vi "ALTS-2015 OPC Write Engine.vi"(8 "error in (no error)":errorcluster, 11 "Delay (ms)":u32=100) -> (0 "error out":errorcluster)   [LabVIEW 2013]
doc: "Copyright © 2005, Soliton Technologies.\nAll rights reserved."
uses:
  Controls/ALTS-2015 OPC Engine Main Options.ctl
  Controls/ALTS-2015 OPC Write Registers.ctl
  Controls/ALTS-2015 OPC Write Global Options.ctl
  Controls/ALTS-2015 OPC Global Options.ctl
  Controls/ALTS-2015 OPC Global Elements.ctl
  Globals/ALTS-2015 OPC Engine Globals.vi
  Controls/ALTS-2015 Safety Logic Cases.ctl
  SLL DAQ Engine/Software/Source Code/Controls/SLL DI Global Options.ctl
  SLL DAQ Engine/Software/Source Code/Controls/SLL List of Digital Inputs.ctl
panel:
  in  "OPC Write Registers":T1=enum."Serial_Flange_Size"
  out "Running Case":T2
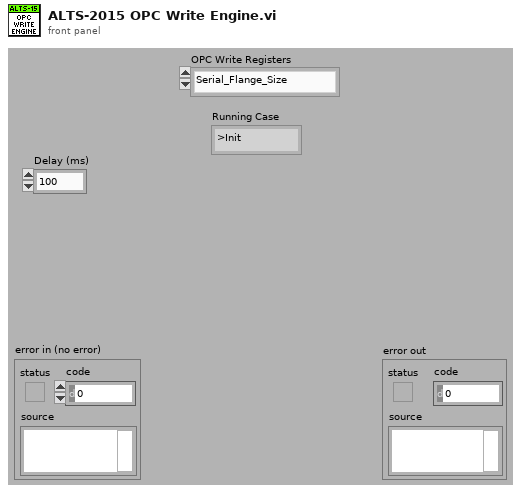
[diagram p1: front panel]
types:
  T1 = typedef "ALTS-2015 OPC Write Registers.ctl" = enum16{"Task_Available_for_Robot", "New_Serial", "Serial_Adapter_Size", "Serial_Displacement_Size", "Serial_Flange_Size", "Serial_Height", "Serial_LoadDecision", "Serial_CartInsert", "Test_Result", "Station_Number", "Rerun", "Invalid_SNo", "PC_ACK_Read_Tags", "No_Test"}
  T2 = typedef "ALTS-2015 OPC Engine Main Options.ctl" = enum16{">Init", ">Safe Mode", ">Poll", ">Error", ">Exit", ">Write", ">Read", ">Restart"}
  T3 = typedef "ALTS-2015 OPC Global Options.ctl" = enum16{"Init", "Write 1", "Read 1", "Write Array", "Read Array", "Clear"}
  T4 = typedef "ALTS-2015 OPC Write Global Options.ctl" = enum16{"Init", "Write Value", "Write Array", "Read Value", "Read Array", "Read All"}
  T5 = cluster{"Channel Order":i32[], "Connection ids":refnum<k13>[], "OPC Write Register Old Value":variant[]}
  T6 = enum16{"Read", "Write", "ReadWrite", "BufferedRead", "BufferedReadWrite"}
  T7 = typedef "ALTS-2015 OPC Global Elements.ctl" = enum16{"OPC - R Error", "OPC - W Error", "OPC - R Restart", "OPC - W Restart", "OPC - R Running", "OPC - W Running"}
  T8 = typedef "SLL List of Digital Inputs.ctl" = enum16{"MSSF", "MSSHC", "MSSMF", "MSSPRM", "MSSR", "PS01TS", "PX03TS", "PX04TS", "PX05TS", "PX06TS", "PX18TS", "READYTS"}
  T9 = typedef "SLL DI Global Options.ctl" = enum16{"Init", "Write Line", "Write Array", "Read Line", "Read Array", "Read Full Status", "Write Full Status"}
  T10 = typedef "ALTS-2015 Safety Logic Cases.ctl" = enum16{"Read S/W EStop", "Read H/W EStop", "Write S/W EStop", "Write H/W EStop", "Read S/W & H/W EStop"}
  T11 = typedef "ALTS-2015 INI Configuration Cluster.ctl" = cluster{"Application":cluster{"Rerun Count":i32, "Workorder No":string, "PLC Scanner":bool}, "Station Details":cluster{"Sensor Name 1":string, "Sensor Name 2":string, "Sensor Name 3":string, "Sensor Name 4":string, "Station1 Enable":bool, "Station2 Enable":bool, "Station3 Enable":bool, "Station4 Enable":bool}, "Database":cluster{"Database Connection Link":path, "Result Procedure":string, "User":string, "Password":string, "Prompt":bool, "Station 1 LT Result DB DSN Path":path, "Station 2 LT Result DB DSN Path":path, "Station 3 LT Result DB DSN Path":path, "Station 4 LT Result DB DSN Path":path, "AirLeakTestResult Procedure":string, "Serial Details Procedure":string}, "Simulation":cluster{"Simulate DAQ Hardware":bool, "Simulate Result DB Write":bool, "Simulate Scanner":bool, "Simulate OPC":bool, "Simulate Serial Details DB":bool, "Simulate Result DB":bool, "Simulate Scanner DB Path":path, "Simulate Serial Details DB Path":path, "Simulate Result DB Path":path}, "Barcode Scanner1":cluster{"Scanner IP":string, "Scanner Port":u16, "#Bytes to Read":i32, "Timeout_ms":i32}, "Barcode Scanner2":cluster{"Enabled?":bool, "Scanner IP":string, "Scanner Port":u16, "#Bytes to Read":i32}}
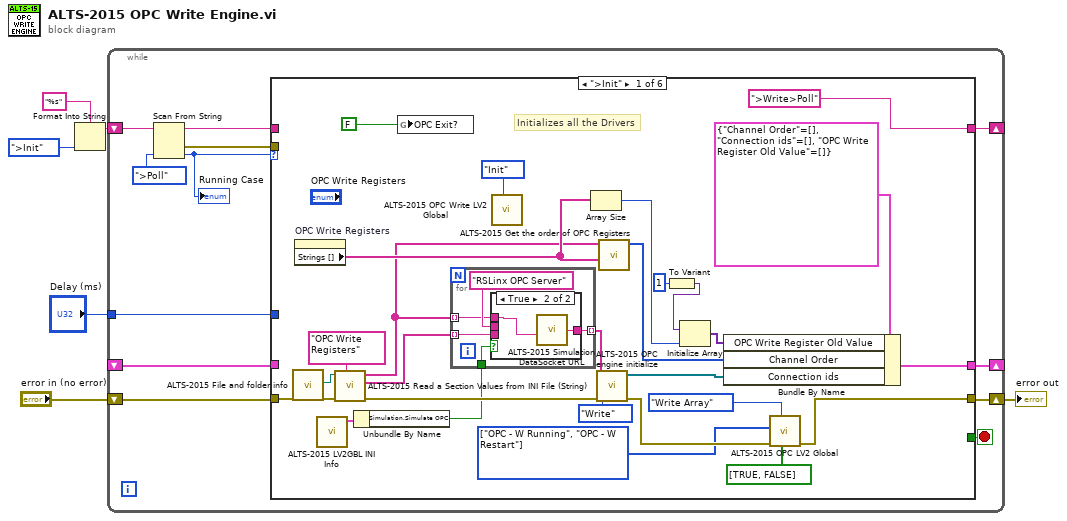
[diagram p0: block diagram]
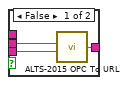
[diagram p2: hidden frame]
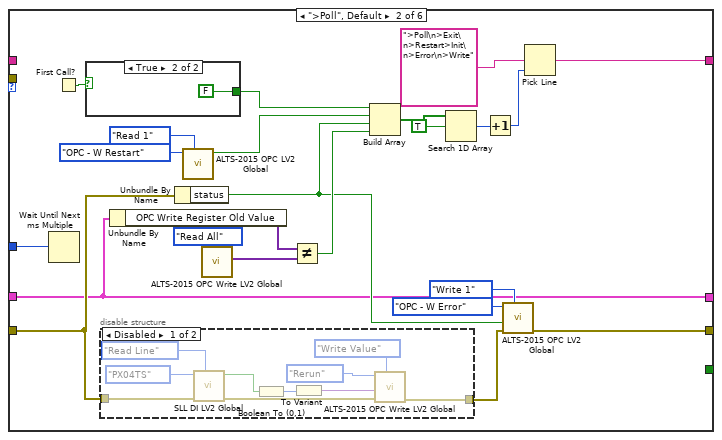
[diagram p3: hidden frame]
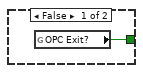
[diagram p5: hidden frame]
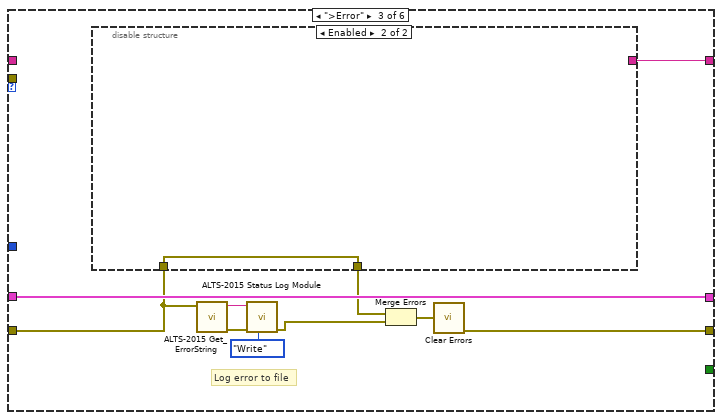
[diagram p6: hidden frame]
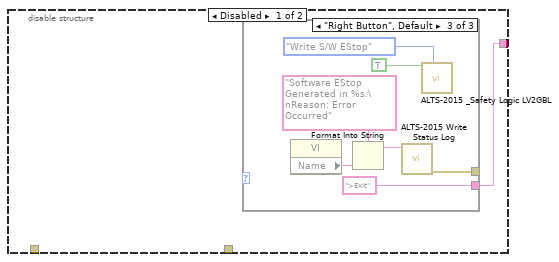
[diagram p7: hidden frame]
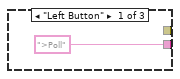
[diagram p8: hidden frame]
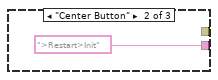
[diagram p9: hidden frame]
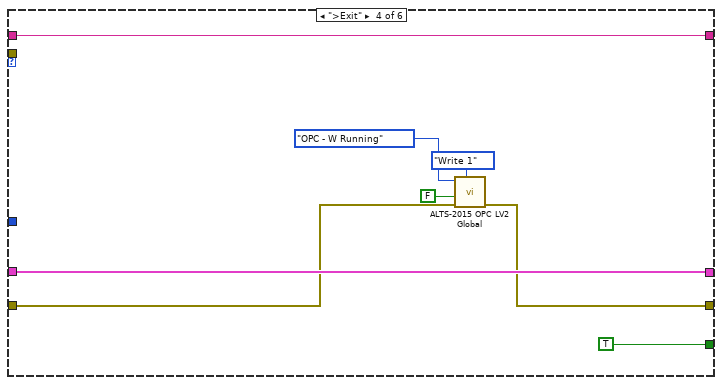
[diagram p10: hidden frame]
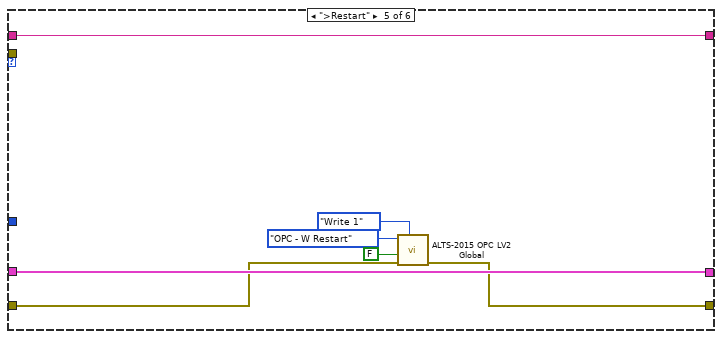
[diagram p11: hidden frame]
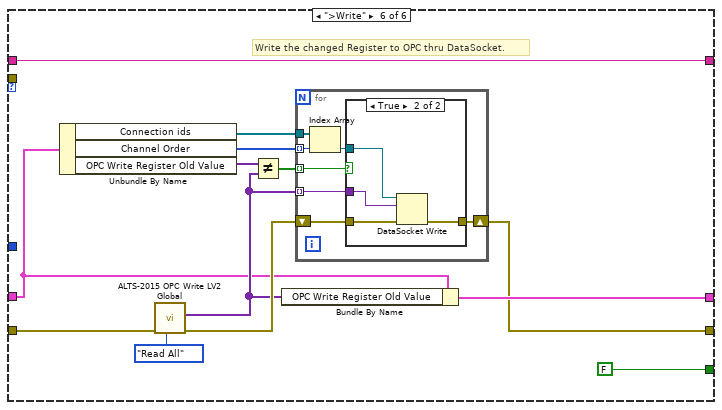
[diagram p12: hidden frame]
diagram:
  n1 = Format Into String(format string="%s", ALTS-2015_OPC_Engine_Main_Options.">Init" ("DAQ Options")) -> (resulting string=w2:string)  [unwired: 2 in, 1 out]
  n2 = while {
    shift-right: [w17] -> w5
    shift-left: "error in (no error)" -> [w18]
    shift-right: [w16] -> _
    shift-left: _ -> [w15]
    shift-right: [w10] -> _
    shift-left: w2 -> [w14]
    tunnel: "Delay (ms)" -> [w8]
    stop <- w9 stop-if-true
    n3 = Scan From String(input string=w14, default 1=ALTS-2015_OPC_Engine_Main_Options.">Poll" ("DAQ Options")) -> (remaining string=w12:string, error out=w11:errorcluster, output 1=w7:T2)  [unwired: 3 in, 1 out]
    "Running Case" <- w7
    n4 = case shown="\">Init\"" w7 {
      tunnel: w18 -> [w43 w59 w95 w116 w125 w141]
      tunnel: [w31 w63 w101 w120 w124 w131] -> w17
      tunnel: [w39 w57 w102 w123 w130 w133] -> w16
      tunnel: w15 -> [_ w57 w102 w123 w130 w132]
      tunnel: w12 -> [_ _ _ w122 w129 w143]
      tunnel: w11 -> [_ _ _ _ _ _]
      tunnel: [">Write>Poll" ("output string") w74 w100 w122 w129 w143] -> w10
      tunnel: [_ _ _ TRUE _ FALSE] -> w9
      tunnel: w8 -> [_ w72 _ _ _ _]
      frame ">Init" {
        w28 = T7[] [enum."OPC - W Running", enum."OPC - W Restart"] items=["OPC - R Error", "OPC - W Error", "OPC - R Restart", "OPC - W Restart", "OPC - R Running", "OPC - W Running"] ("Elements Array")
        # "Initializes all the Drivers"
        n5 = call "ALTS-2015 File and folder info.vi"("error in (no error)"=w43) -> ("INI file path"=w42:path, "error out"=w38:errorcluster)  [unwired: 9 in, 8 out]
        n6 = property on="OPC Write Registers" class="Enum (strict)"() -> ("Strings []"=w23:string[])  [unwired: 2 in, 2 out]
        n7 = call "ALTS-2015 LV2GBL INI Info.vi"() -> ("Configuration Cluster Out"=w21:T11)  [unwired: 10 in, 1 out]
        n8 = call "ALTS-2015 Read a Section Values from INI File (String).vi"("Section"="OPC Write Registers", "error in (no error)"=w38, "INI File Path"=w42) -> ("error out"=w45:errorcluster, "Key Values"=w29:string[], "Key Names"=w19:string[])  [unwired: 6 in]
        n9 = Unbundle By Name(w21) -> ("Simulation.Simulate OPC"=w20:bool)
        n10 = global write "ALTS-2015 OPC Engine Globals.vi" "OPC Exit?"(FALSE ("DAQ Exit?")) -> ()
        n11 = for {
          tunnel: w29 -> [w51] mode=indexing
          tunnel: [w50] -> w30 mode=indexing
          tunnel: w20 -> [w48]
          tunnel: w19 -> [w47] mode=indexing
          n12 = case shown="True" w48 {
            tunnel: w51 -> [w54 _]
            tunnel: [w53 w56] -> w50
            tunnel: "RSLinx OPC Server" ("Server Name") -> [w52 _]
            tunnel: w47 -> [_ w55]
            frame False {
              n13 = call "ALTS-2015 OPC To URL.vi"("Item Name"=w54, "Server Name"=w52) -> ("URL"=w53:string)  [unwired: 4 in]
            }
            frame True {
              n14 = call "ALTS-2015 Simulation DataSocket URL.vi"("Item Name"=w55) -> ("URL"=w56:string)  [unwired: 5 in]
            }
          }
        }
        n15 = call "ALTS-2015 OPC Write LV2 Global.vi"("Options"=ALTS-2015_OPC_Write_Global_Options."Init") -> ()  [unwired: 8 in, 3 out]
        n16 = Array Size(array=w23) -> (size(s)=w22:i32)
        n17 = call "ALTS-2015 OPC engine initialize.vi"("error in (no error)"=w45, "mode"=T6."Write", "URLs"=w30) -> ("error out"=w32:errorcluster, "Connection ids"=w40:refnum<k13>[])  [unwired: 7 in]
        n18 = call "ALTS-2015 Get the order of OPC Registers.vi"("Register Names - Enum"=w23, "Register Names - INI"=w19) -> ("Channel Order"=w37:i32[])  [unwired: 8 in, 1 out]
        n19 = To Variant(anything=1) -> (Variant=w24:variant)
        n20 = Initialize Array(w24, w22) -> (w25:variant[])
        n21 = Bundle By Name(cluster=T5 {"Channel Order"=[], "Connection ids"=[], "OPC Write Register Old Value"=[]} ("Data Cluster"), "OPC Write Register Old Value"=w25, "Channel Order"=w37, "Connection ids"=w40) -> (w39:T5)
        n22 = call "ALTS-2015 OPC LV2 Global.vi"("Status Array In"=bool[] [TRUE, FALSE], "Option"=ALTS-2015_OPC_Global_Options."Write Array", "error in (no error)"=w32, "Elements Array"=w28) -> ("error out"=w31:errorcluster)  [unwired: 5 in, 2 out]
      }
      frame ">Poll", Default {
        n23 = Wait Until Next ms Multiple(millisecond multiple=w72) -> ()  [unwired: 1 out]
        n24 = First Call?() -> (First Call?: T/F=w60:bool)
        n25 = case shown="True" w60 {
          tunnel: [w91 FALSE ("OPC Exit?")] -> w73
          frame False {
            n26 = global read "ALTS-2015 OPC Engine Globals.vi" "OPC Exit?"() -> (w91:bool)
          }
          frame True {
          }
        }
        n27 = disable-structure shown="Disabled" {
          disable-tunnel: w59 -> [w87 w90]
          disable-tunnel: [w80 w90] -> w58
          frame Disabled {
            n28 = call "SLL DI LV2 Global.vi"("Option"=SLL_DI_Global_Options."Read Line", "error in (no error)"=w87, "DI Channel Name"=SLL_List_of_Digital_Inputs."PX04TS" ("DI Channel Name 2")) -> ("error out"=w86:errorcluster, "Digital Line Status"=w82:bool)  [unwired: 5 in, 2 out]
            n29 = Boolean To (0,1)(Boolean=w82) -> (0, 1=w83:i16)
            n30 = To Variant(anything=w83) -> (Variant=w81:variant)
            n31 = call "ALTS-2015 OPC Write LV2 Global.vi"("Options"=ALTS-2015_OPC_Write_Global_Options."Write Value", "error in (no error)"=w86, "OPC value"=w81, "OPC Write Register"=ALTS-2015_OPC_Write_Registers."Rerun") -> ("error out"=w80:errorcluster)  [unwired: 5 in, 2 out]
          }
          frame Enabled {
          }
        }
        n32 = Unbundle By Name(w57) -> ("OPC Write Register Old Value"=w69:variant[])
        n33 = Unbundle By Name(w59) -> ("status"=w64:bool)
        n34 = call "ALTS-2015 OPC LV2 Global.vi"("Option"=ALTS-2015_OPC_Global_Options."Read 1", "Elements"=ALTS-2015_OPC_Global_Elements."OPC - W Restart") -> ("Status Out"=w67:bool)  [unwired: 7 in, 2 out]
        n35 = call "ALTS-2015 OPC Write LV2 Global.vi"("Options"=ALTS-2015_OPC_Write_Global_Options."Read All") -> ("OPC Read Register Array Value"=w70:variant[])  [unwired: 8 in, 2 out]
        n36 = Not Equal?(x=w69, y=w70) -> (x != y?=w68:bool)
        n37 = Build Array(w73, w67, w64, w68) -> (w78:bool[])
        n38 = Search 1D Array(1D array=w78, element=TRUE) -> (index of element=w76:i32)  [unwired: 1 in]
        n39 = Increment(x=w76) -> (x+1=w75:i32)
        n40 = call "ALTS-2015 OPC LV2 Global.vi"("Option"=ALTS-2015_OPC_Global_Options."Write 1", "error in (no error)"=w58, "Status In"=w64, "Elements"=ALTS-2015_OPC_Global_Elements."OPC - W Error") -> ("error out"=w63:errorcluster)  [unwired: 5 in, 2 out]
        n41 = Pick Line(multi-line string=">Poll\n>Exit\n>Restart>Init\n>Error\n>Write", line index=w75) -> (output string=w74:string)  [unwired: 1 in]
      }
      frame ">Error" {
        # "Log error to file"
        n42 = disable-structure shown="Enabled" {
          disable-tunnel: [w105 _] -> w100
          disable-tunnel: w95 -> [w104 w115]
          disable-tunnel: [w103 w115] -> w94
          frame Disabled {
            n43 = case shown="\"Right Button\", Default" {
              selector: _ -> [_ _ _]
              tunnel: [">Poll" ("format string") ">Restart>Init" ("format string") ">Exit" ("format string")] -> w105
              tunnel: [_ _ w108] -> _
              frame "Left Button" {
              }
              frame "Center Button" {
              }
              frame "Right Button", Default {
                n44 = property class="VI"() -> ("Name"=w110:string)  [unwired: 2 in, 2 out]
                n45 = Format Into String(format string="Software EStop Generated in %s.\nReason: Error Occurred" ("Status Input"), w110) -> (resulting string=w111:string)  [unwired: 2 in, 1 out]
                n46 = call "ALTS-2015 Write Status Log.vi"("Status Input"=w111) -> ("error out"=w108:errorcluster)  [unwired: 10 in]
                n47 = call "ALTS-2015 _Safety Logic LV2GBL.vi"("Options"=ALTS-2015_Safety_Logic_Cases."Write S/W EStop", "EStop In"=TRUE) -> ()  [unwired: 6 in, 4 out]
              }
            }
          }
          frame Enabled {
          }
        }
        n48 = call "ALTS-2015 Get_ErrorString.vi"("Incoming Error"=w95) -> ("error out"=w96:errorcluster, "Message"=w98:string)  [unwired: 9 in]
        n49 = call "ALTS-2015 Status Log Module.vi"("Options"=enum16{"Init", "Write", "Close"}."Write", "error in"=w96, "Text to  Log"=w98) -> ("error out"=w97:errorcluster)  [unwired: 8 in]
        n50 = Merge Errors(w94, w97) -> (w93:errorcluster)
        n51 = call <vilib>:"Clear Errors.vi"("error in (no error)"=w93) -> ("error out"=w101:errorcluster)  [unwired: 6 in]
      }
      frame ">Exit" {
        n52 = call "ALTS-2015 OPC LV2 Global.vi"("Option"=ALTS-2015_OPC_Global_Options."Write 1", "error in (no error)"=w116, "Status In"=FALSE, "Elements"=ALTS-2015_OPC_Global_Elements."OPC - W Running") -> ("error out"=w120:errorcluster)  [unwired: 5 in, 2 out]
      }
      frame ">Restart" {
        n53 = call "ALTS-2015 OPC LV2 Global.vi"("Option"=ALTS-2015_OPC_Global_Options."Write 1", "error in (no error)"=w125, "Status In"=FALSE, "Elements"=ALTS-2015_OPC_Global_Elements."OPC - W Restart") -> ("error out"=w124:errorcluster)  [unwired: 5 in, 2 out]
      }
      frame ">Write" {
        # "Write the changed Register to OPC thru DataSocket."
        n54 = Unbundle By Name(w132) -> ("Connection ids"=w137:refnum<k13>[], "Channel Order"=w136:i32[], "OPC Write Register Old Value"=w139:variant[])
        n55 = call "ALTS-2015 OPC Write LV2 Global.vi"("Options"=ALTS-2015_OPC_Write_Global_Options."Read All", "error in (no error)"=w141) -> ("error out"=w135:errorcluster, "OPC Read Register Array Value"=w134:variant[])  [unwired: 7 in, 1 out]
        n56 = Not Equal?(x=w139, y=w134) -> (x != y?=w138:bool[])
        n57 = Bundle By Name(cluster=w132, "OPC Write Register Old Value"=w134) -> (w133:T5)
        n58 = for {
          tunnel: w138 -> [w149] mode=indexing
          tunnel: w137 -> [w145]
          tunnel: w136 -> [w146] mode=indexing
          tunnel: w134 -> [w150] mode=indexing
          shift-right: [w147] -> w131
          shift-left: w135 -> [w148]
          n59 = Index Array(array=w145, index=w146) -> (element=w144:refnum<k13>)
          n60 = case shown="True" w149 {
            tunnel: w144 -> [_ w155]
            tunnel: w150 -> [_ w154]
            tunnel: w148 -> [w151 w153]
            tunnel: [w151 w152] -> w147
            frame False {
            }
            frame True {
              n61 = DataSocket Write(8:w153, 10:w154, 11:w155) -> (0:w152:errorcluster)  [unwired: 1 in, 2 out]
            }
          }
        }
      }
    }
  }
  "error out" <- w5
